vi "CarWashClient.vi"() -> ()   [LabVIEW 2024]
uses:
  purchase_selection_state1.ctl
  main_wash_state.ctl
panel:
  out "timer":dbl
  out "Car Wash Type":string
  in  "stop":bool
  in  "Car Wash Indicators":enum32{"Purchase Selection"}(tab)
  out "Under Body Wash":bool
  out "Soap Application":bool
  out "Main High Pressure Wash":bool
  out "Clear Water Rinse":bool
  out "Air Dry":bool
  in  "Vehicle Out of Position":bool
  in  "Car Wash Simulation Switches":enum32{"Purchase Selection"}(tab)
  in  "Air Dry\nPosition\nSwitch":bool
  in  "Main Wash\nPosition\nSwitch":bool
  in  "Under Body \nWash Position \nSwitch":bool
  in  "Purchase Selection":enum32{"Purchase Selection"}(tab)
  in  "Deluxe Wash":bool
  in  "Economy Wash":bool
  # "Client"
  # "Step 1: Select an option\nof car wash"
  # "Step 3: Observe the indicators"
  # "Car Wash Indicators"
  # "Illustration"
  # "Purchase Selection"
  # "Step 2: Click the simulation \nswitches"
  # "Car Wash Simulation Switches"
  # "1.\tUnderbody Wash – 10 seconds \n2.\tSoap Application – 5 seconds \n3.\tMain High-Pressure Wash – 5 seconds \n4.\tClear Water rinse – 5 seconds \n5.\tAir Dry Cycle – 10 seconds"
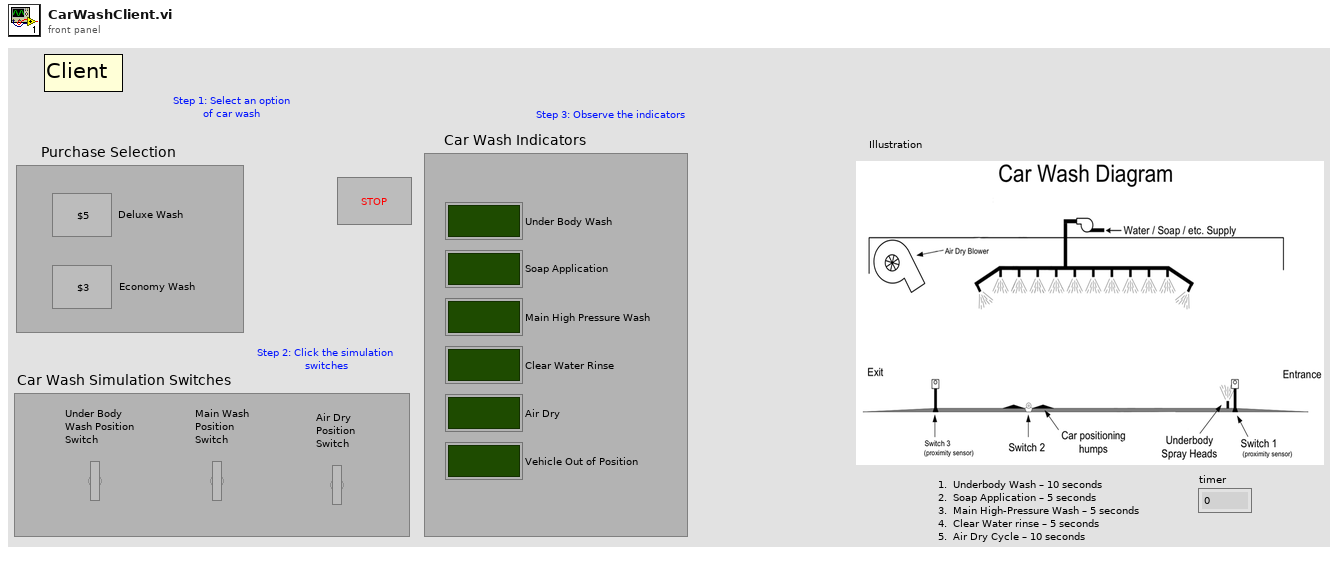
[diagram p1: front panel]
types:
  T1 = typedef "purchase_selection_state1.ctl" = enum16{"init", "wait", "underbody wash", "main wash", "air dry", "log", "end"}
  T2 = enum8{"Enabled", "Disabled", "Disabled and Grayed Out"}
  T3 = typedef "main_wash_state.ctl" = enum16{"init", "soap application", "main high pressure wash", "clear water rinse", "end"}
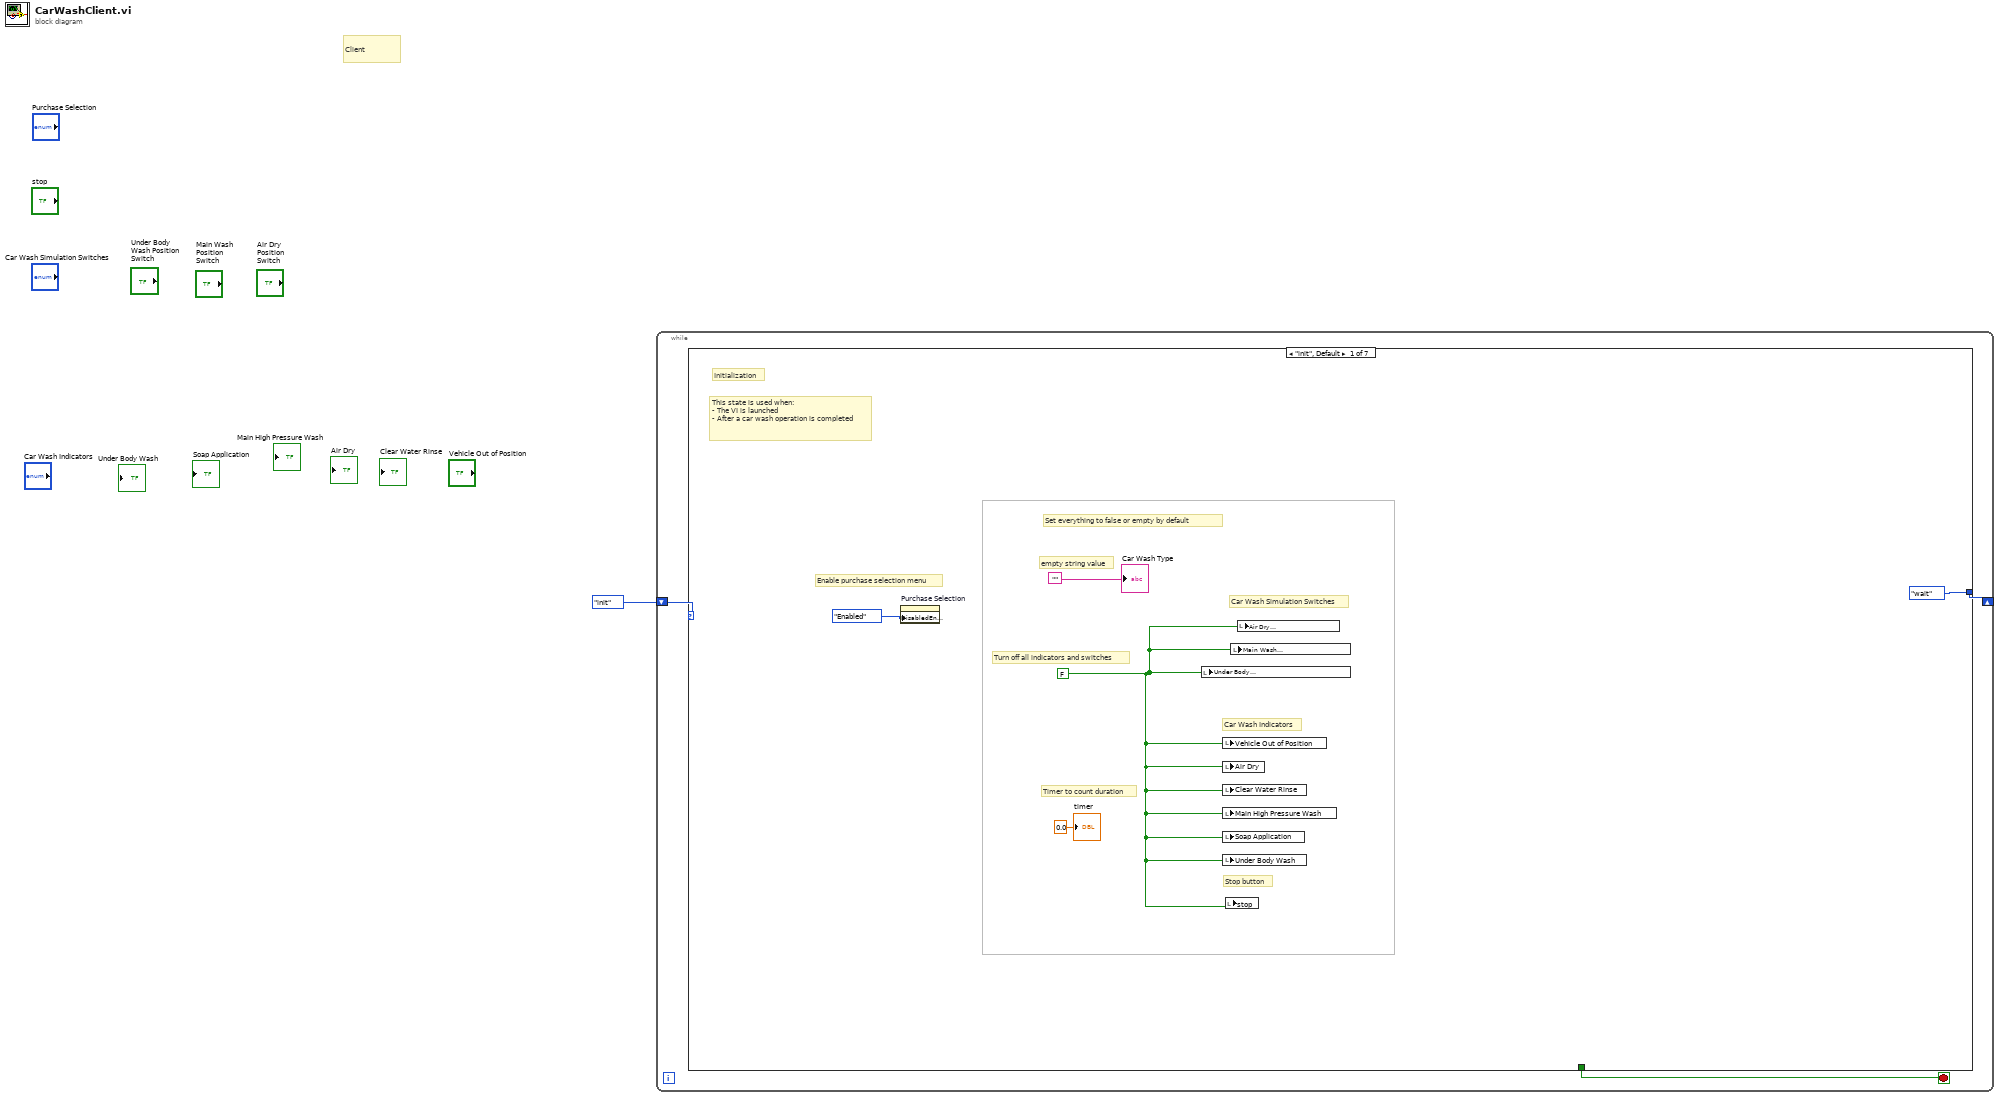
[diagram p0: block diagram]
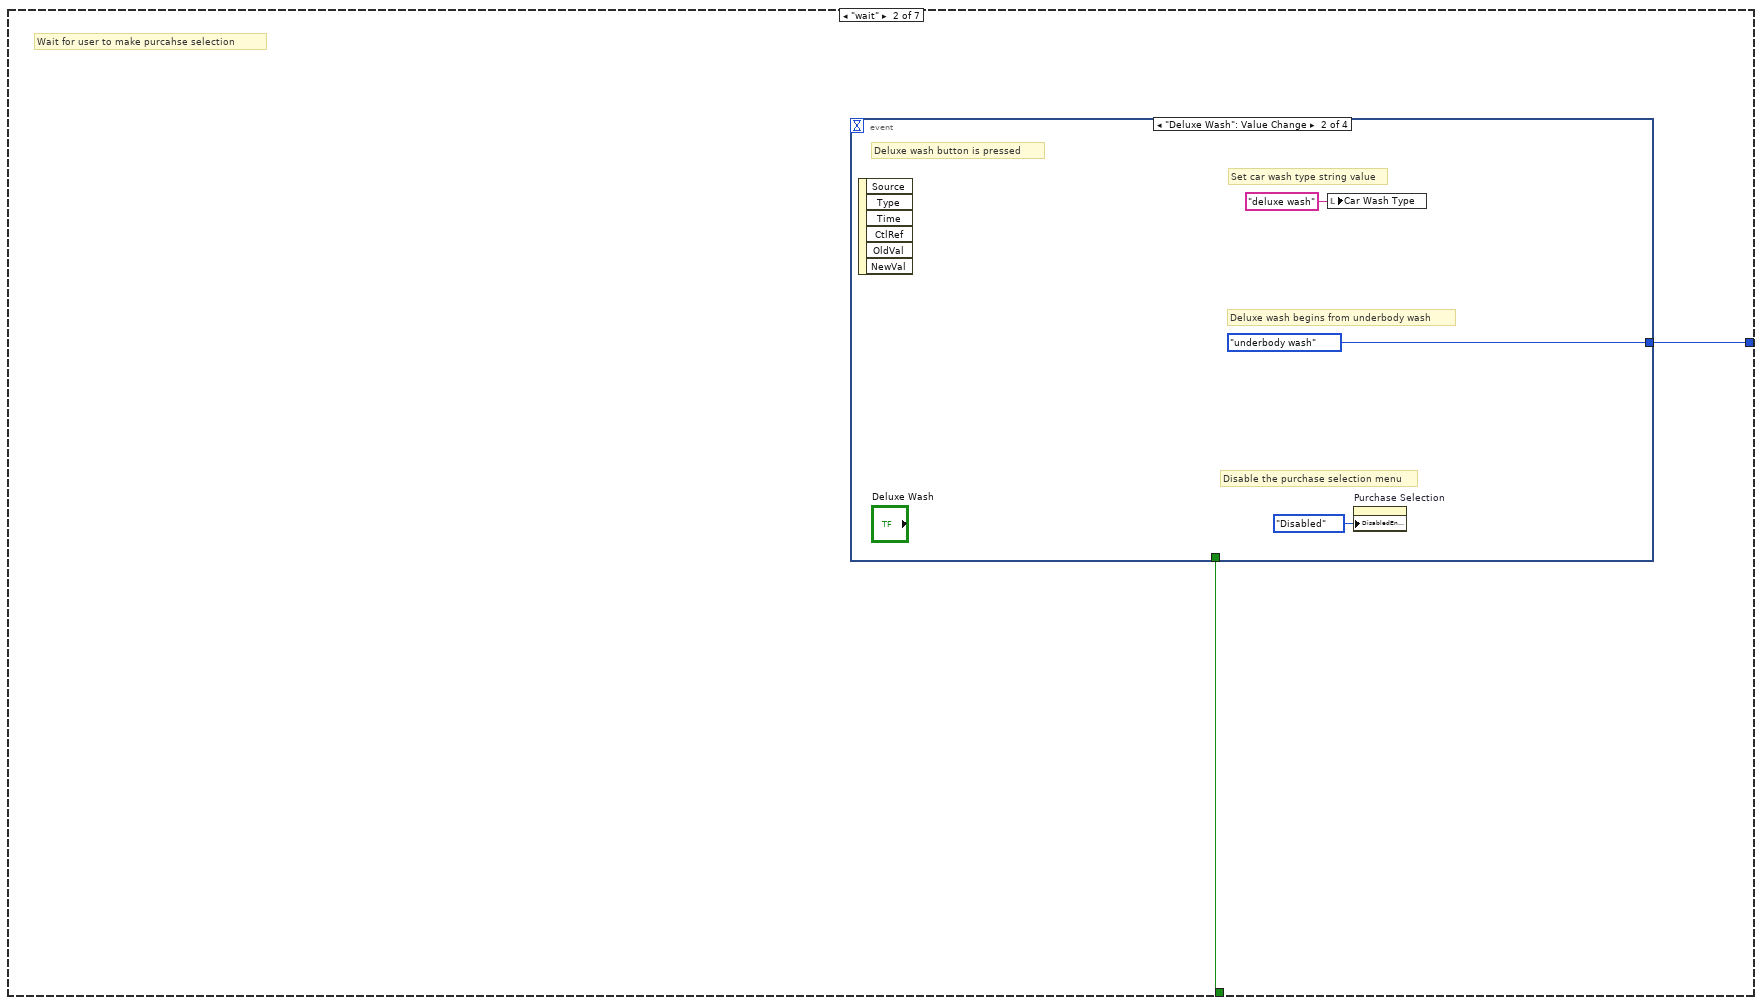
[diagram p2: hidden frame]
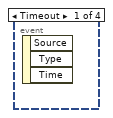
[diagram p3: hidden frame]
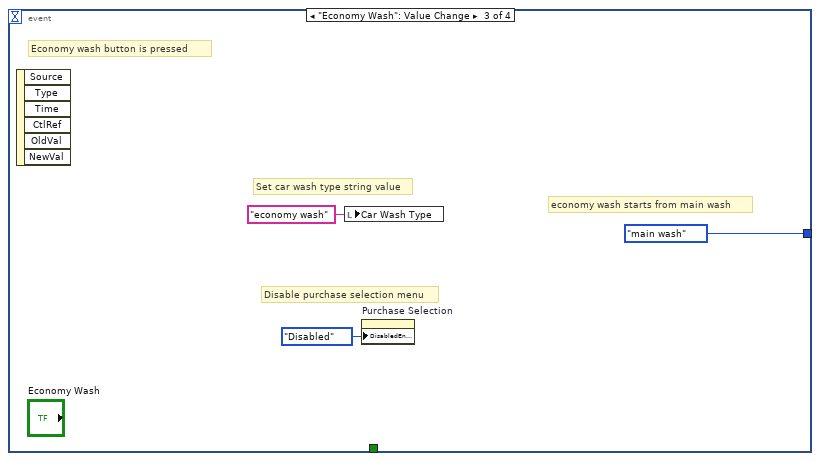
[diagram p4: hidden frame]
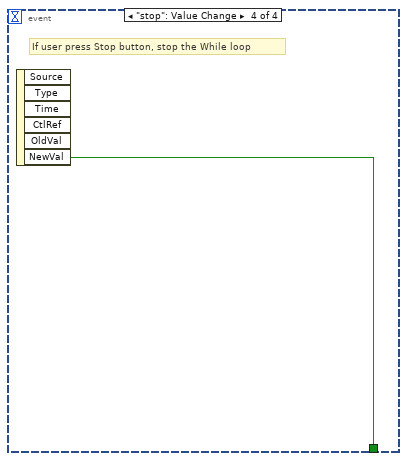
[diagram p5: hidden frame]
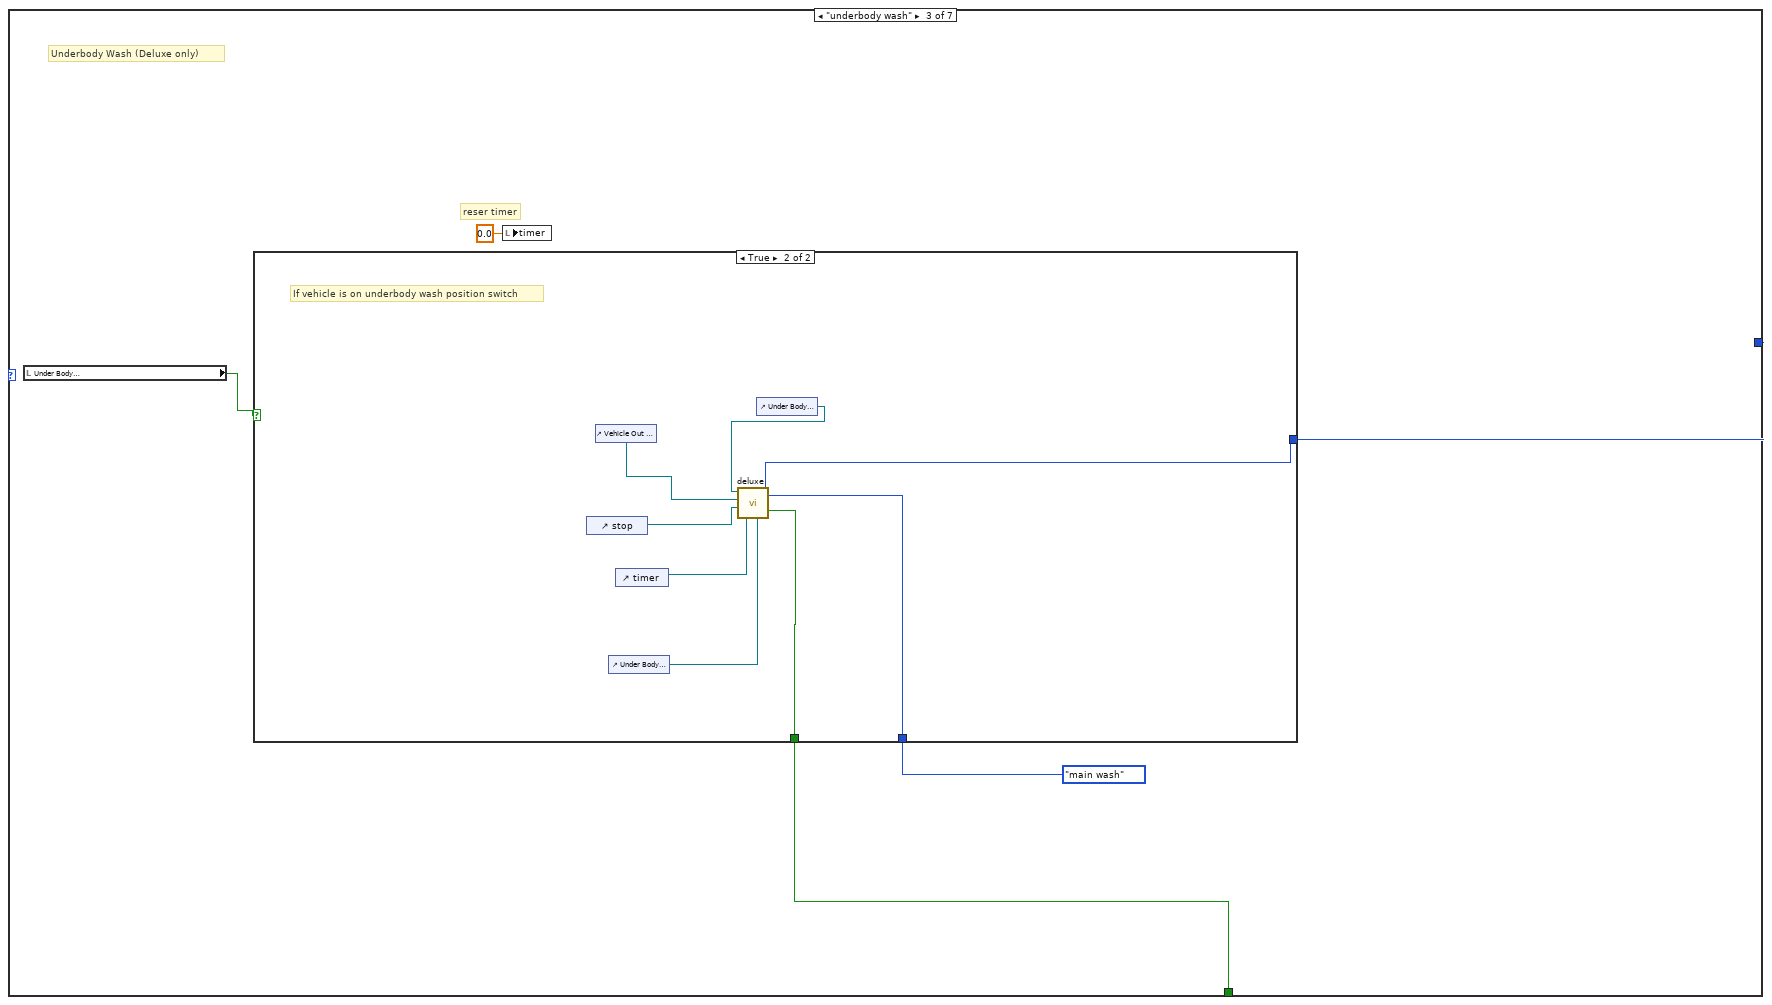
[diagram p6: hidden frame]
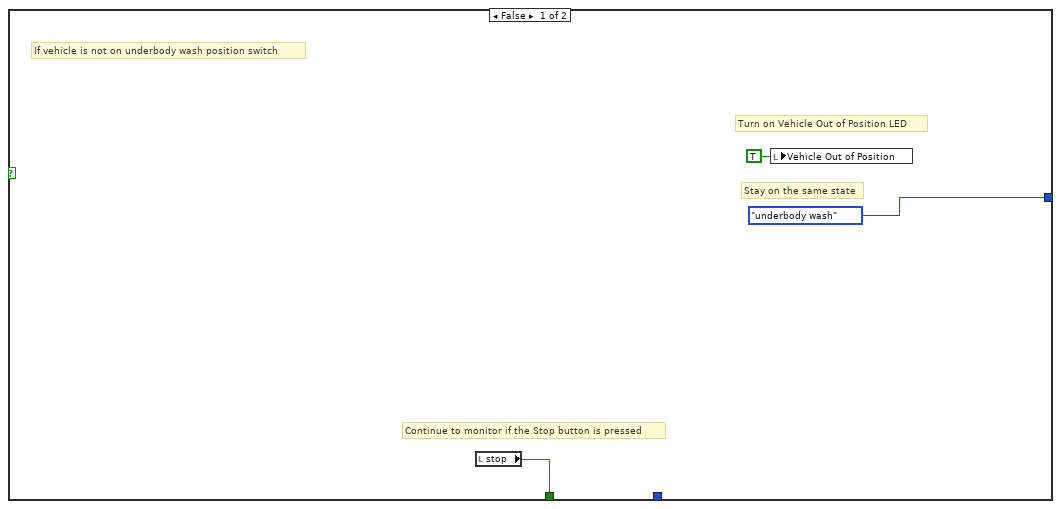
[diagram p7: hidden frame]
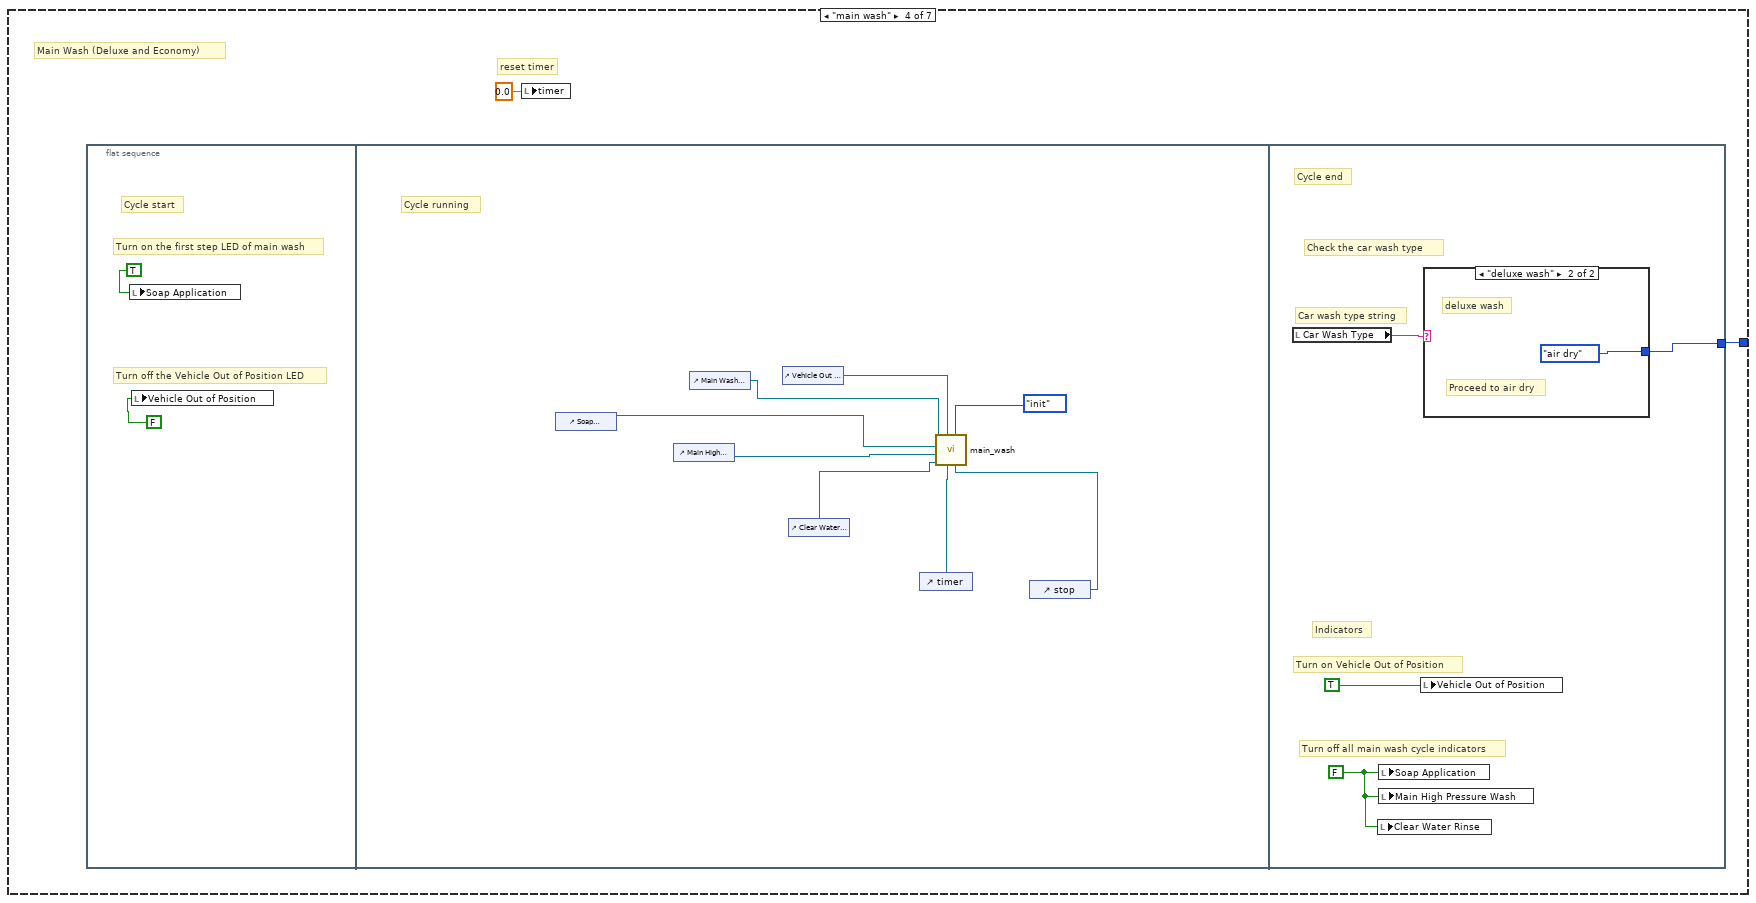
[diagram p8: hidden frame]
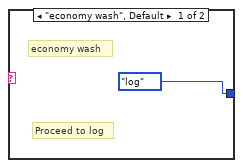
[diagram p9: hidden frame]
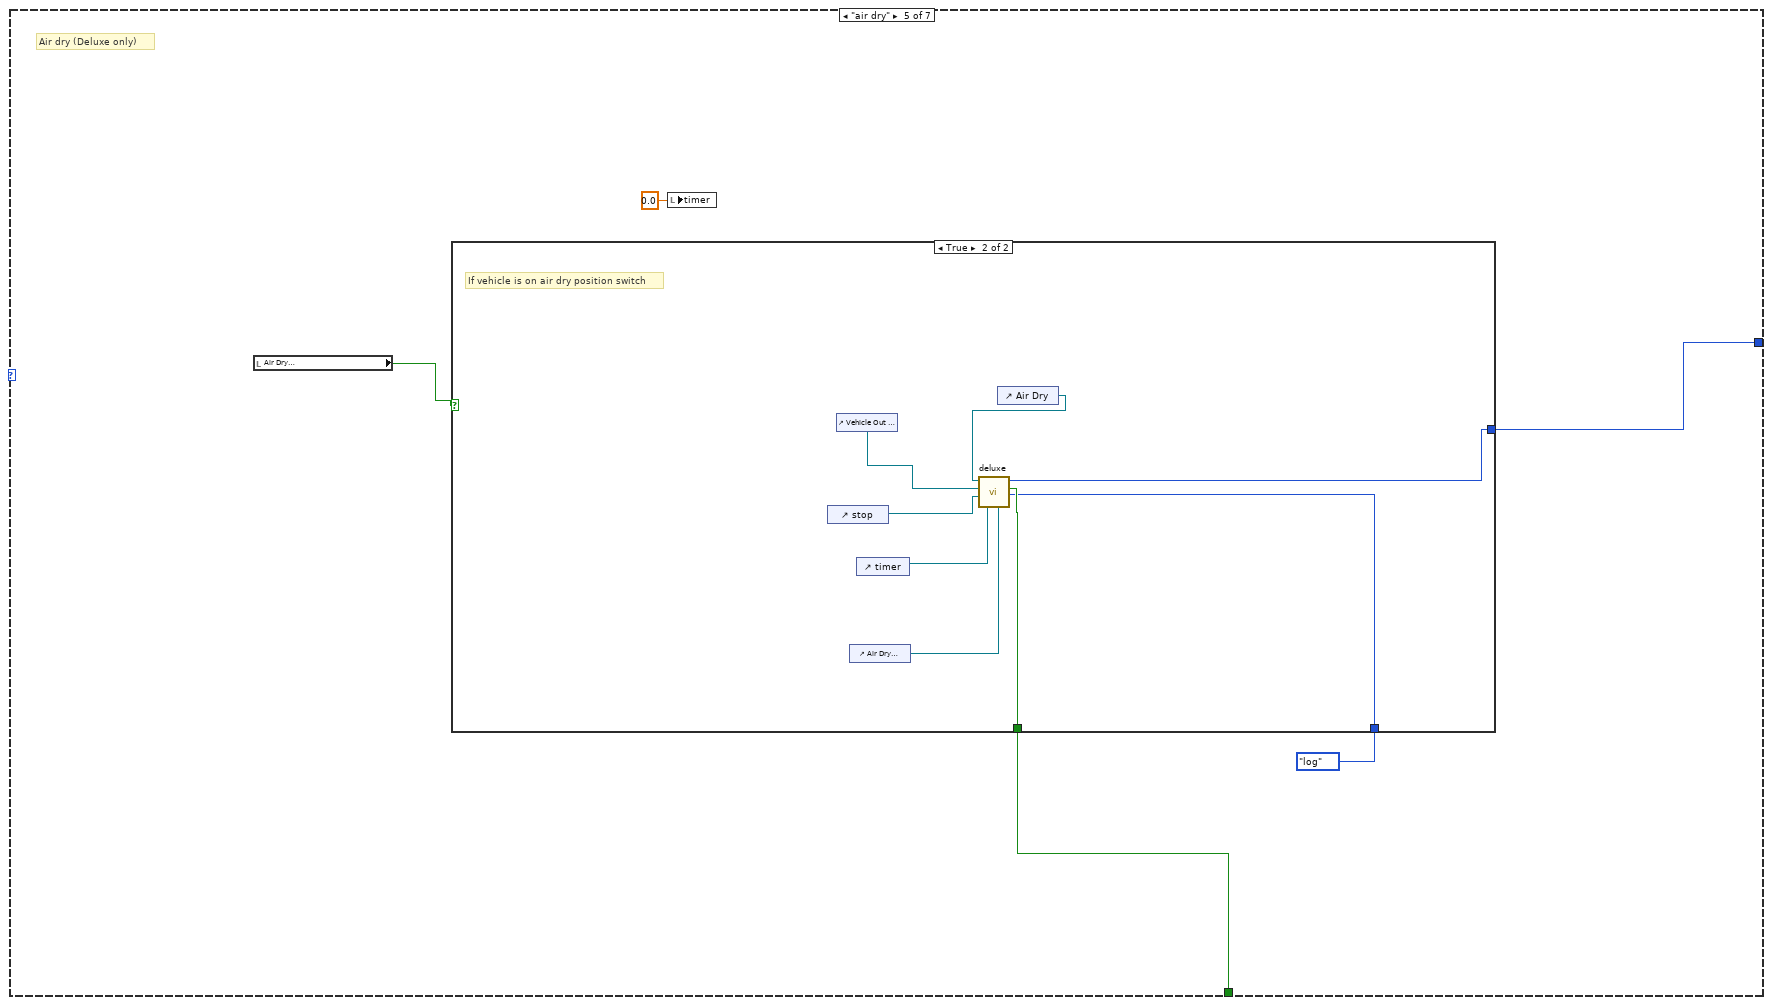
[diagram p10: hidden frame]
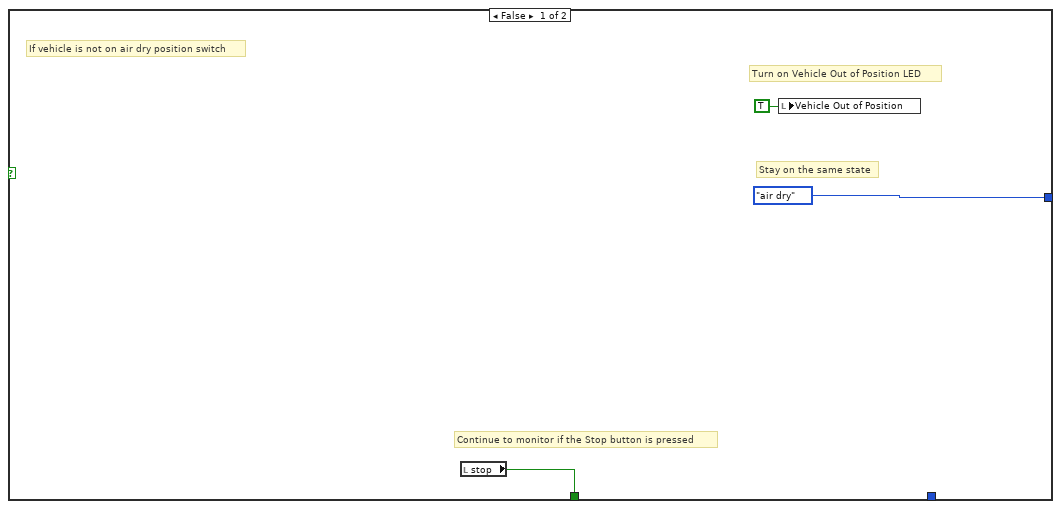
[diagram p11: hidden frame]
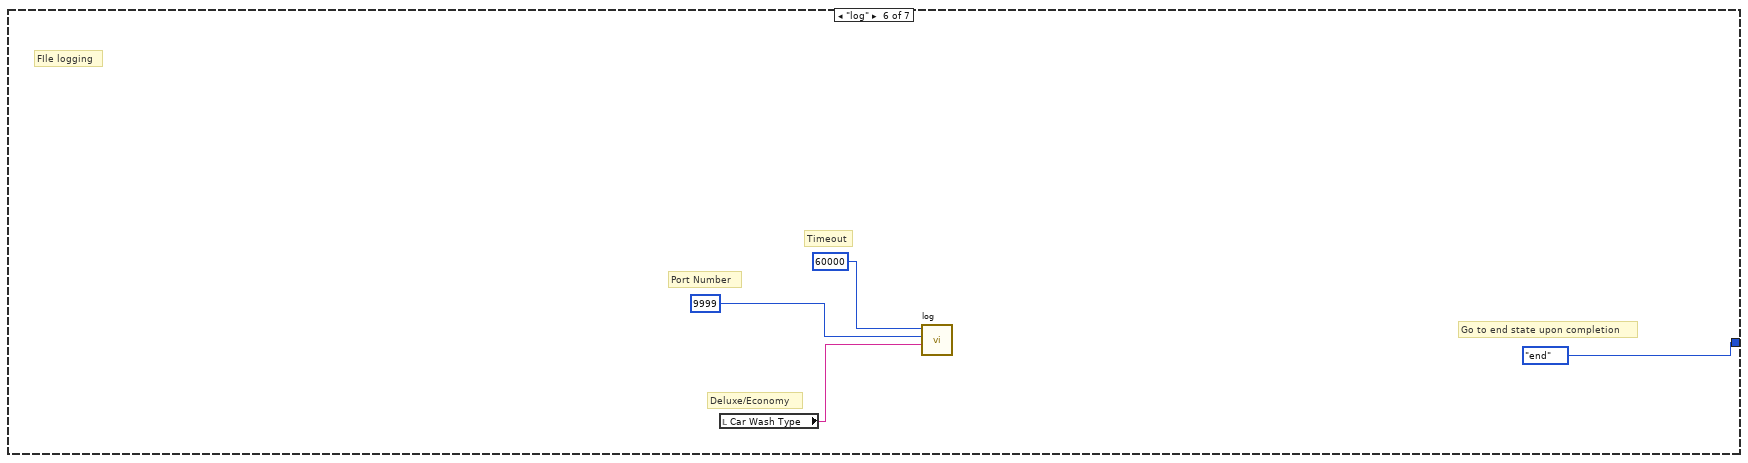
[diagram p12: hidden frame]
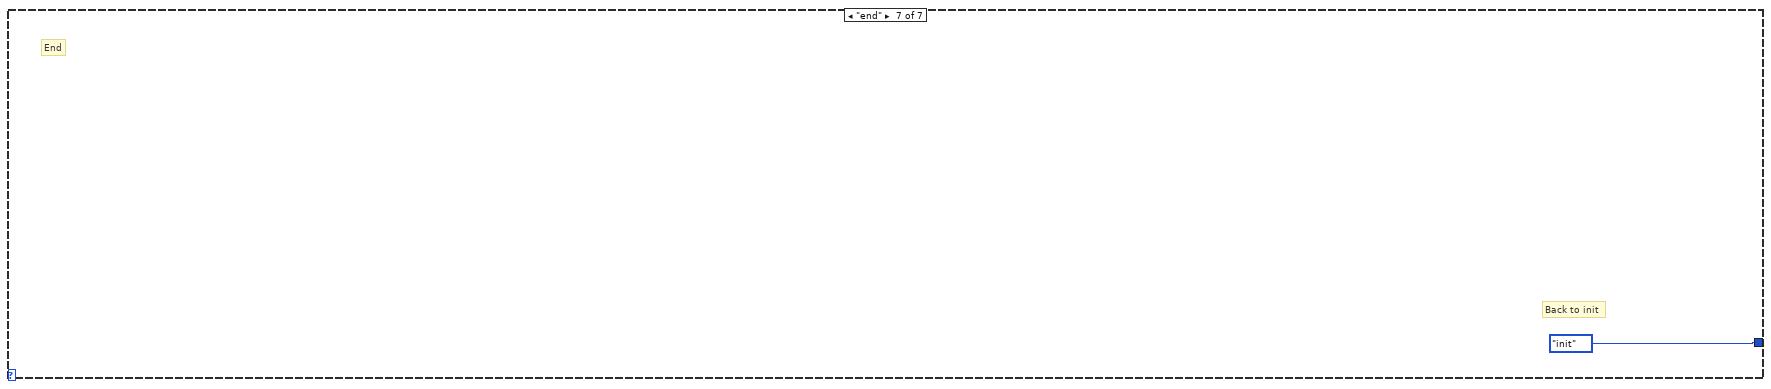
[diagram p13: hidden frame]
diagram:
  # "Client"
  n1 = while {
    shift-right: [w3] -> _
    shift-left: purchase_selection_state1."init" -> [w4]
    stop <- w2 stop-if-true
    n2 = case shown="\"init\", Default" w4 {
      tunnel: [purchase_selection_state1."wait" w11 w22 w35 w55 purchase_selection_state1."end" purchase_selection_state1."init"] -> w3
      tunnel: [_ w10 w20 _ w54 _ _] -> w2
      frame "init", Default {
        w5 = FALSE
        # "Turn off all indicators and switches"
        # "This state is used when:\n- The VI is launched\n- After a car wash operation is completed"
        # "Stop button"
        # "Timer to count duration"
        # "empty string value"
        # "Enable purchase selection menu"
        # "Set everything to false or empty by default"
        # "Car Wash Indicators"
        # "Car Wash Simulation Switches"
        # "Initialization"
        n3 = property on="Purchase Selection" class="TabCtl (strict)"("DisabledEnum"=T2."Enabled" ("Disabled")) -> ()  [unwired: 2 in, 2 out]
        n4 = local write "Under Body \nWash Position \nSwitch"(w5) -> ()
        n5 = local write "Vehicle Out of Position"(w5) -> ()
        n6 = local write "Air Dry"(w5) -> ()
        n7 = local write "Clear Water Rinse"(w5) -> ()
        n8 = local write "Main High Pressure Wash"(w5) -> ()
        n9 = local write "Soap Application"(w5) -> ()
        n10 = local write "Under Body Wash"(w5) -> ()
        n11 = local write "stop"(w5) -> ()
        n12 = local write "Main Wash\nPosition\nSwitch"(w5) -> ()
        n13 = local write "Air Dry\nPosition\nSwitch"(w5) -> ()
        "Car Wash Type" <- ""
        "timer" <- 0.0 ("timer")
      }
      frame "wait" {
        # "Wait for user to make purcahse selection"
        n14 = event shown="[1] \"Deluxe Wash\": Value Change" {
          selector: _ -> [_ _ _ _]
          dyn-events: _ -> [_ _ _ _]
          timeout: _ -> [_ _ _ _]
          tunnel: [_ purchase_selection_state1."underbody wash" purchase_selection_state1."main wash" _] -> w11
          tunnel: [_ _ _ w18] -> w10
          event Timeout {
            n15 = event-data() -> ()  [unwired: 1 in, 3 out]
          }
          event "Deluxe Wash": Value Change {
            # "Disable the purchase selection menu"
            # "Deluxe wash begins from underbody wash"
            # "Set car wash type string value"
            # "Deluxe wash button is pressed"
            n16 = event-data() -> ()  [unwired: 1 in, 6 out]
            n17 = local write "Car Wash Type"("deluxe wash" ("Car Wash Type")) -> ()
            n18 = property on="Purchase Selection" class="TabCtl (strict)"("DisabledEnum"=T2."Disabled" ("Disabled")) -> ()  [unwired: 2 in, 2 out]
          }
          event "Economy Wash": Value Change {
            # "Set car wash type string value"
            # "economy wash starts from main wash"
            # "Disable purchase selection menu"
            # "Economy wash button is pressed"
            n19 = event-data() -> ()  [unwired: 1 in, 6 out]
            n20 = local write "Car Wash Type"("economy wash" ("Car Wash Type")) -> ()
            n21 = property on="Purchase Selection" class="TabCtl (strict)"("DisabledEnum"=T2."Disabled" ("Disabled")) -> ()  [unwired: 2 in, 2 out]
          }
          event "stop": Value Change {
            # "If user press Stop button, stop the While loop"
            n22 = event-data() -> ("NewVal"=w18:bool)  [unwired: 1 in, 5 out]
          }
        }
      }
      frame "underbody wash" {
        # "reser timer"
        # "Underbody Wash (Deluxe only)"
        n23 = local read "Under Body \nWash Position \nSwitch"() -> (w23:bool)
        n24 = case shown="True" w23 {
          tunnel: [purchase_selection_state1."underbody wash" w28] -> w22
          tunnel: [w24 w29] -> w20
          tunnel: purchase_selection_state1."main wash" -> [_ w27]
          frame False {
            # "Continue to monitor if the Stop button is pressed"
            # "Stay on the same state"
            # "Turn on Vehicle Out of Position LED"
            # "If vehicle is not on underbody wash position switch"
            n25 = local read "stop"() -> (w24:bool)
            n26 = local write "Vehicle Out of Position"(TRUE ("Vehicle Out of Position")) -> ()
          }
          frame True {
            # "If vehicle is on underbody wash position switch"
            n27 = control-ref of="stop"() -> (w32:refnum<vi>)
            n28 = control-ref of="Vehicle Out of Position"() -> (w33:refnum<vi>)
            n29 = control-ref of="Under Body \nWash Position \nSwitch"() -> (w30:refnum<vi>)
            n30 = control-ref of="timer"() -> (w31:refnum<vi>)
            n31 = control-ref of="Under Body Wash"() -> (w34:refnum<vi>)
            n32 = call "deluxe.vi"("Current cycle switch"=w30, "timer"=w31, "Next state in"=w27, "Stop"=w32, "Vehicle out of position"=w33, "Current cycle indicator"=w34) -> ("stop"=w29:bool, "Next state out"=w28:T1)  [unwired: 4 in]
          }
        }
        n33 = local write "timer"(0.0 ("timer")) -> ()
      }
      frame "main wash" {
        # "reset timer"
        # "Main Wash (Deluxe and Economy)"
        n34 = flat-sequence {
          tunnel: [w49] -> w35
          frame #0 {
            # "Turn off the Vehicle Out of Position LED"
            # "Turn on the first step LED of main wash"
            # "Cycle start"
            n35 = local write "Soap Application"(TRUE ("Under Body Wash")) -> ()
            n36 = local write "Vehicle Out of Position"(FALSE ("Under Body Wash")) -> ()
          }
          frame #1 {
            # "Cycle running"
            n37 = control-ref of="Soap Application"() -> (w44:refnum<vi>)
            n38 = control-ref of="Main High Pressure Wash"() -> (w43:refnum<vi>)
            n39 = control-ref of="Main Wash\nPosition\nSwitch"() -> (w39:refnum<vi>)
            n40 = control-ref of="Vehicle Out of Position"() -> (w45:refnum<vi>)
            n41 = control-ref of="Clear Water Rinse"() -> (w42:refnum<vi>)
            n42 = control-ref of="timer"() -> (w41:refnum<vi>)
            n43 = control-ref of="stop"() -> (w40:refnum<vi>)
            n44 = call "main_wash.vi"("Stop"=w40, "Main wash state"=main_wash_state."init", "timer"=w41, "Vehicle out of position"=w45, "Clear water rinse"=w42, "Main high pressure wash"=w43, "Soap application"=w44, "Cycle Switch"=w39) -> ()  [unwired: 4 in]
          }
          frame #2 {
            w47 = FALSE ("Under Body Wash")
            # "Turn off all main wash cycle indicators"
            # "Turn on Vehicle Out of Position"
            # "Car wash type string"
            # "Indicators"
            # "Check the car wash type"
            # "Cycle end"
            n45 = local read "Car Wash Type"() -> (w48:string)
            n46 = local write "Clear Water Rinse"(w47) -> ()
            n47 = local write "Soap Application"(w47) -> ()
            n48 = local write "Main High Pressure Wash"(w47) -> ()
            n49 = local write "Vehicle Out of Position"(TRUE ("Under Body Wash")) -> ()
            n50 = case shown="\"deluxe wash\"" w48 {
              tunnel: [purchase_selection_state1."log" purchase_selection_state1."air dry"] -> w49
              frame "economy wash", Default {
                # "Proceed to log"
                # "economy wash"
              }
              frame "deluxe wash" {
                # "Proceed to air dry"
                # "deluxe wash"
              }
            }
          }
        }
        n51 = local write "timer"(0.0 ("timer")) -> ()
      }
      frame "air dry" {
        # "Air dry (Deluxe only)"
        n52 = local read "Air Dry\nPosition\nSwitch"() -> (w56:bool)
        n53 = case shown="True" w56 {
          tunnel: [purchase_selection_state1."air dry" w66] -> w55
          tunnel: [w58 w68] -> w54
          tunnel: purchase_selection_state1."log" -> [_ w67]
          frame False {
            # "Continue to monitor if the Stop button is pressed"
            # "Stay on the same state"
            # "Turn on Vehicle Out of Position LED"
            # "If vehicle is not on air dry position switch"
            n54 = local read "stop"() -> (w58:bool)
            n55 = local write "Vehicle Out of Position"(TRUE ("Vehicle Out of Position")) -> ()
          }
          frame True {
            # "If vehicle is on air dry position switch"
            n56 = control-ref of="stop"() -> (w63:refnum<vi>)
            n57 = control-ref of="Vehicle Out of Position"() -> (w64:refnum<vi>)
            n58 = control-ref of="Air Dry\nPosition\nSwitch"() -> (w61:refnum<vi>)
            n59 = control-ref of="timer"() -> (w62:refnum<vi>)
            n60 = control-ref of="Air Dry"() -> (w65:refnum<vi>)
            n61 = call "deluxe.vi"("Current cycle switch"=w61, "timer"=w62, "Next state in"=w67, "Stop"=w63, "Vehicle out of position"=w64, "Current cycle indicator"=w65) -> ("stop"=w68:bool, "Next state out"=w66:T1)  [unwired: 4 in]
          }
        }
        n62 = local write "timer"(0.0 ("timer")) -> ()
      }
      frame "log" {
        # "Go to end state upon completion"
        # "Deluxe/Economy"
        # "Timeout"
        # "Port Number"
        # "FIle logging"
        n63 = local read "Car Wash Type"() -> (w69:string)
        n64 = call "log.vi"("Car Wash Type"=w69, "remote port or service name"=u16 9999, "timeout ms (60000)"=60000) -> ()  [unwired: 9 in]
      }
      frame "end" {
        # "End"
        # "Back to init"
      }
    }
  }
